vi "Actor Core.vi"(8 "error in":errorcluster, 11 "Samples in":refnum<class "Samples.lvclass">) -> (0 "error out":errorcluster, 3 "Actor out":refnum<class "Actor.lvclass">)   [LabVIEW 2015, in "AMS UI.lvlib" / "Samples.lvclass"]
doc: "(<B>Filename</B>: Actor Framework.lvlib:Actor.lvclass:Actor Core.vi)\n\nReceives messages to the actor, reacts to them, and initiates any error handling that may shut the actor down.\n\nDescendant classes may override this VI to append parallel tasks for the actor to complete while it handles messages. Overrides use the Call Parent Method node."
uses:
  Samples.lvclass
  <vilib>/ActorFramework/Actor/Actor.lvclass
  <vilib>/ActorFramework/Message Enqueuer/Message Enqueuer.lvclass/Message Enqueuer.ctl
  <vilib>/ActorFramework/Report Error Msg/Report Error Msg.lvclass/Report Error Msg.ctl
  <vilib>/ActorFramework/Message Enqueuer/Enqueue.vi
  <vilib>/ActorFramework/Message Priority Queue/Priority Enqueue.vi
  <vilib>/ActorFramework/Message Enqueuer/Message Enqueuer.lvclass
  Samples Messages/Indicate Samples Msg/Indicate Samples Msg.lvclass
  <vilib>/ActorFramework/Report Error Msg/Report Error Msg.lvclass
  AMS Gas Actor/AMS Gas Actor.lvclass
panel:
  out "Numeric Control":i32
  in  "Sample In 2":bool caption="Sample In"
  in  "Ti Cathode 2":i8 caption="Ti Cathode" min=-1 max=39
  in  "Name 2":string caption="Name"
  in  "Sample In 5":bool caption="Sample In"
  in  "Ti Cathode 5":i8 caption="Ti Cathode" min=-1 max=39
  in  "Name 5":string caption="Name"
  in  "Sample In 4":bool caption="Sample In"
  in  "Ti Cathode 4":i8 caption="Ti Cathode" min=-1 max=39
  in  "Name 4":string caption="Name"
  in  "Sample In 3":bool caption="Sample In"
  in  "Ti Cathode 3":i8 caption="Ti Cathode" min=-1 max=39
  in  "Name 3":string caption="Name"
  in  "Sample In 1":bool caption="Sample In"
  in  "Ti Cathode 1":i8 caption="Ti Cathode" min=-1 max=39
  in  "Name 1":string caption="Name"
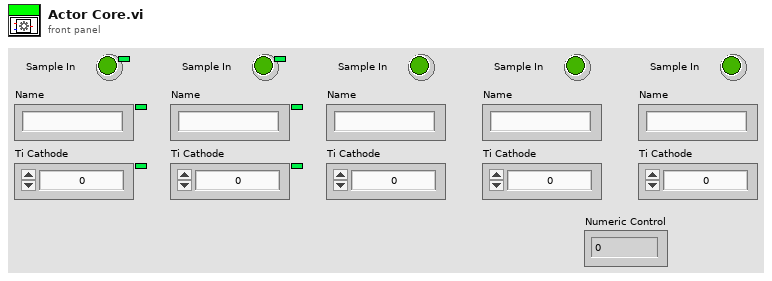
[diagram p1: front panel]
types:
  T1 = cluster{"Sample In":refnum<vi>, "Ti Cathode":refnum<vi>, "Name":refnum<vi>}
  T2 = cluster{"Sample In":refnum<vi>, "Ti Cathode":refnum<vi>, "Name":refnum<vi>}[]
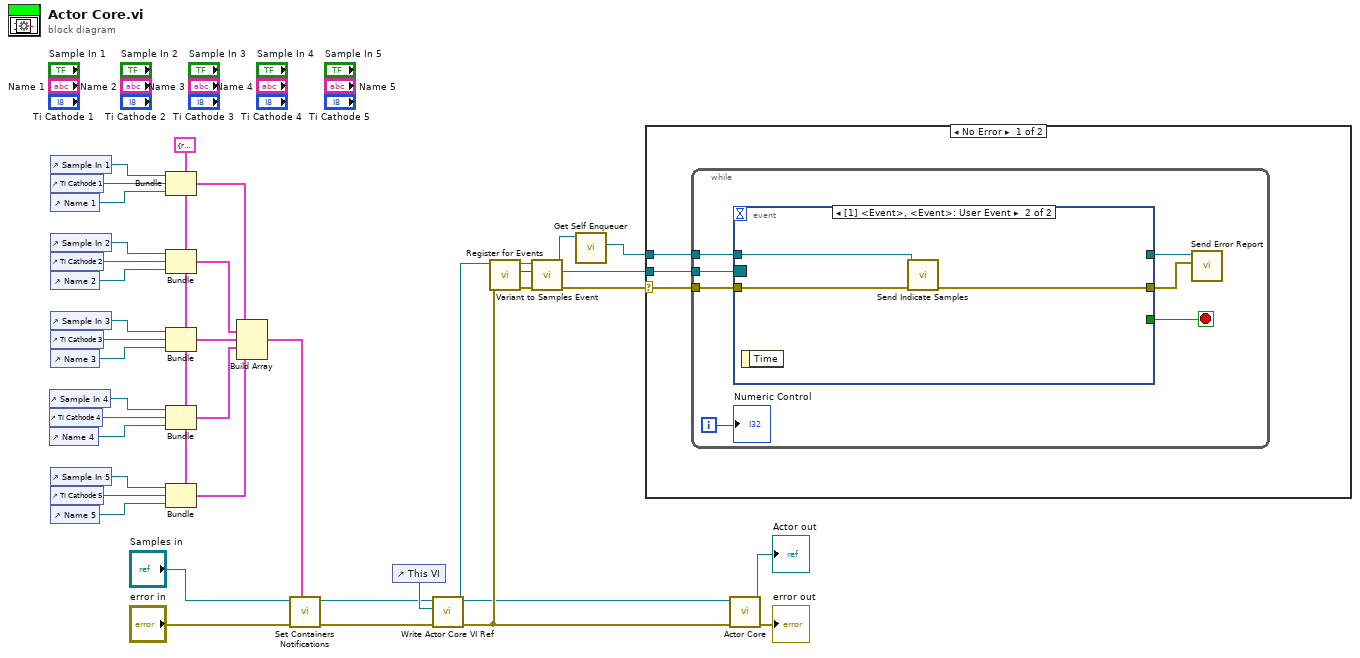
[diagram p0: block diagram]
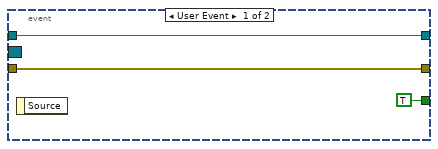
[diagram p2: hidden frame]
diagram:
  w11 = T1 {"Sample In"=refnum, "Ti Cathode"=refnum, "Name"=refnum} ("output cluster")
  n1 = control-ref of="Sample In 4"() -> (w17:refnum<vi>)
  n2 = control-ref of="Ti Cathode 4"() -> (w16:refnum<vi>)
  n3 = control-ref of="Name 4"() -> (w15:refnum<vi>)
  n4 = control-ref of="Sample In 1"() -> (w26:refnum<vi>)
  n5 = control-ref of="Ti Cathode 1"() -> (w25:refnum<vi>)
  n6 = control-ref of="Name 1"() -> (w24:refnum<vi>)
  n7 = control-ref of="Sample In 2"() -> (w23:refnum<vi>)
  n8 = control-ref of="Ti Cathode 2"() -> (w22:refnum<vi>)
  n9 = control-ref of="Name 2"() -> (w21:refnum<vi>)
  n10 = control-ref of="Sample In 3"() -> (w20:refnum<vi>)
  n11 = control-ref of="Ti Cathode 3"() -> (w19:refnum<vi>)
  n12 = control-ref of="Name 3"() -> (w18:refnum<vi>)
  n13 = control-ref of="Sample In 5"() -> (w14:refnum<vi>)
  n14 = control-ref of="Ti Cathode 5"() -> (w13:refnum<vi>)
  n15 = control-ref of="Name 5"() -> (w12:refnum<vi>)
  n16 = Bundle(cluster=w11, "Sample In"=w26, "Ti Cathode"=w25, "Name"=w24) -> (w10:T1)
  n17 = Bundle(cluster=w11, "Sample In"=w23, "Ti Cathode"=w22, "Name"=w21) -> (w6:T1)
  n18 = Bundle(cluster=w11, "Sample In"=w20, "Ti Cathode"=w19, "Name"=w18) -> (w9:T1)
  n19 = Bundle(cluster=w11, "Sample In"=w17, "Ti Cathode"=w16, "Name"=w15) -> (w7:T1)
  n20 = Bundle(cluster=w11, "Sample In"=w14, "Ti Cathode"=w13, "Name"=w12) -> (w8:T1)
  n21 = Build Array(w10, w6, w9, w7, w8) -> (w1:T2)
  n22 = call "Set Containers Notifications.vi"("Ref Array"=w1, "error in (no error)"="error in", "Samples in"="Samples in") -> ("error out"=w2:errorcluster, "Samples out"=w4:refnum<class "Samples.lvclass">)  [unwired: 7 in]
  n23 = control-ref of="This VI"() -> (w30:refnum<vi>)
  n24 = call "Write Actor Core VI Ref.vi"("error in (no error)"=w2, "Actor Core VI Ref"=w30, "AMS Gas Actor in"=w4) -> ("error out"=w31:errorcluster, "AMS Gas Actor out"=w29:refnum<class "Samples.lvclass">)  [unwired: 7 in]
  n25 = call-dynamic "Register for Events.vi"("error in (no error)"=w31, "Samples in"=w29) -> ("error out"=w36:errorcluster, "Event Registration Refnum"=w34:variant, "Samples out"=w35:refnum<class "Samples.lvclass">)  [unwired: 7 in]
  n26 = call "Variant to Samples Event.vi"("error in (no error)"=w36, "Variant"=w34, "Samples in"=w35) -> ("error out"=w28:errorcluster, "Event Registration Refnum"=w27:refnum<event-registration>, "Samples out"=w33:refnum<class "Samples.lvclass">)  [unwired: 6 in]
  n27 = call-dynamic "Get Self Enqueuer.vi"("eActor in"=w33) -> ("Actor Framework:Message Enqueuer"=w32:refnum<class "Message Enqueuer.lvclass">)  [unwired: 9 in, 1 out]
  n28 = case shown="No Error" w28 {
    selector: w28 -> [w40 _]
    tunnel: w27 -> [w41 _]
    tunnel: w32 -> [w39 _]
    frame No Error {
      n29 = while {
        tunnel: w41 -> [w48]
        tunnel: w40 -> [w47]
        tunnel: w39 -> [w45]
        i -> [w42]
        stop <- w46 stop-if-true
        n30 = event shown="[1] <Event>, <Event>: User Event" {
          selector: w48 -> [_ _]
          dyn-events: _ -> [_ _]
          timeout: _ -> [_ _]
          tunnel: w47 -> [w50 w54]
          tunnel: [w50 w53] -> w44
          tunnel: [TRUE _] -> w46
          tunnel: w45 -> [w49 w52]
          tunnel: [w49 _] -> w43
          event User Event {
            n31 = event-data() -> ()  [unwired: 1 in, 1 out]
          }
          event User Event {
            n32 = event-data() -> ()  [unwired: 1 in, 1 out]
            n33 = call "Send Indicate Samples.vi"("error in (no error)"=w54, "Message Enqueuer"=w52) -> ("error out"=w53:errorcluster)  [unwired: 8 in, 1 out]
          }
        }
        n34 = call <vilib>:"Send Error Report.vi"("Error From Sender"=w44, "Message Enqueuer"=w43) -> ()  [unwired: 9 in, 1 out]
        "Numeric Control" <- w42
      }
    }
    frame Error {
    }
  }
  n35 = call-parent "Actor Core.vi"("error in"=w31, "Actor in"=w29) -> ("error out"=→"error out":errorcluster, "Actor out"=→"Actor out":refnum<class "Actor.lvclass">)  [unwired: 8 in]
